vi "Delta estimate.vi"() -> ()   [LabVIEW 2021]
panel:
  out "x/y":dbl
  in  "Tc":dbl=42.5
  out "Delta 0":dbl format="%#_6p"
  out "Delta/Delta0":dbl
  in  "H":dbl=42.5
  in  "Hc2":dbl=42.5
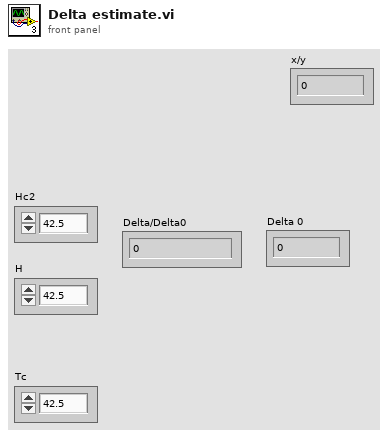
[diagram p1: front panel]
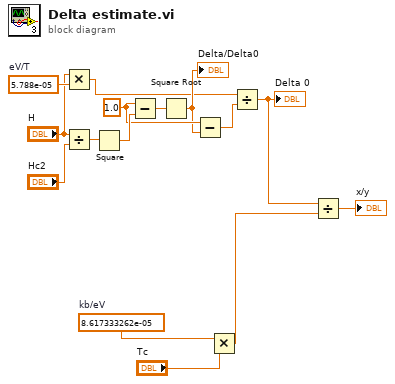
[diagram p0: block diagram]
diagram:
  w5 = 8.617333262e-05  # kb/eV
  w9 = 1.0 ("x")
  w11 = 5.788e-05  # eV/T
  n1 = Multiply(x="H", y=w11) -> (x*y=w7:dbl)
  n2 = Divide(x="H", y="Hc2") -> (x/y=w14:dbl)
  n3 = Square(x=w14) -> (x^2=w13:dbl)
  n4 = Subtract(x=w9, y=w13) -> (x-y=w12:dbl)
  n5 = Square Root(x=w12) -> (sqrt(x)=w8:dbl)
  "Delta/Delta0" <- w8
  n6 = Subtract(x=w9, y=w8) -> (x-y=w6:dbl)
  n7 = Multiply(x=w5, y="Tc") -> (x*y=w2:dbl)
  n8 = Divide(x=w7, y=w6) -> (x/y=w3:dbl)
  "Delta 0" <- w3
  n9 = Divide(x=w3, y=w2) -> (x/y=→"x/y":dbl)
